vi "Read Setting.vi"(8 "error in (no error)":errorcluster, 11 "Update I16 in":refnum<class "Update I16.lvclass">) -> (0 "error out":errorcluster, 2 "Setting":i16, 3 "Update I16 out":refnum<class "Update I16.lvclass">)   [LabVIEW 2014, in "Update I16.lvclass"]
uses:
  Update I16.lvclass
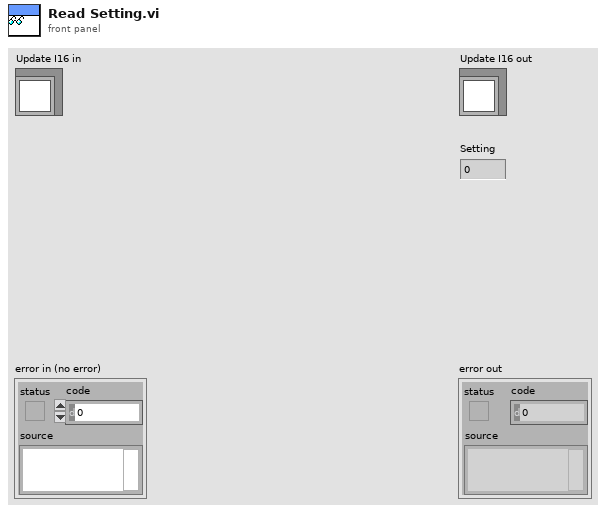
[diagram p1: front panel]
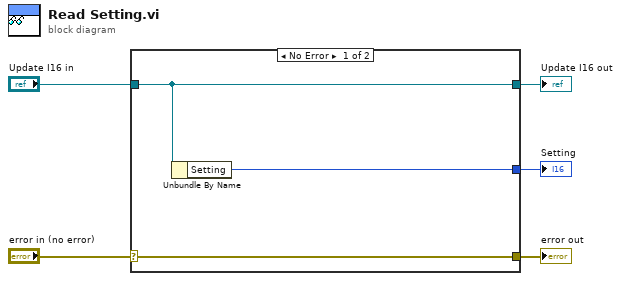
[diagram p0: block diagram]
diagram:
  n1 = case shown="No Error" "error in (no error)" {
    selector: "error in (no error)" -> [w8 w9]
    tunnel: [w8 w9] -> w4
    tunnel: [w7 w10] -> w2
    tunnel: "Update I16 in" -> [w7 w10]
    tunnel: [w6 _] -> w1
    frame No Error {
      n2 = Unbundle By Name(w7) -> ("Setting"=w6:i16)
    }
    frame Error {
    }
  }
  "error out" <- w4
  "Update I16 out" <- w2
  "Setting" <- w1
